vi "VIP_Pre-Install Custom Action.vi"(10 "Variant":variant) -> (0 "error out":errorcluster)   [LabVIEW 2020]
uses:
  <userlib>/_OpenG.lib/file/file.llb/openg_file.lvlib
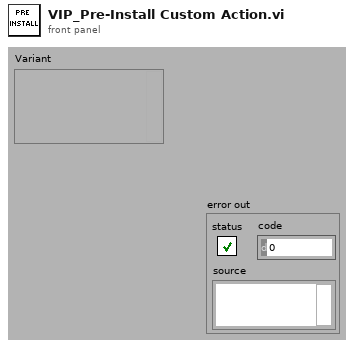
[diagram p1: front panel]
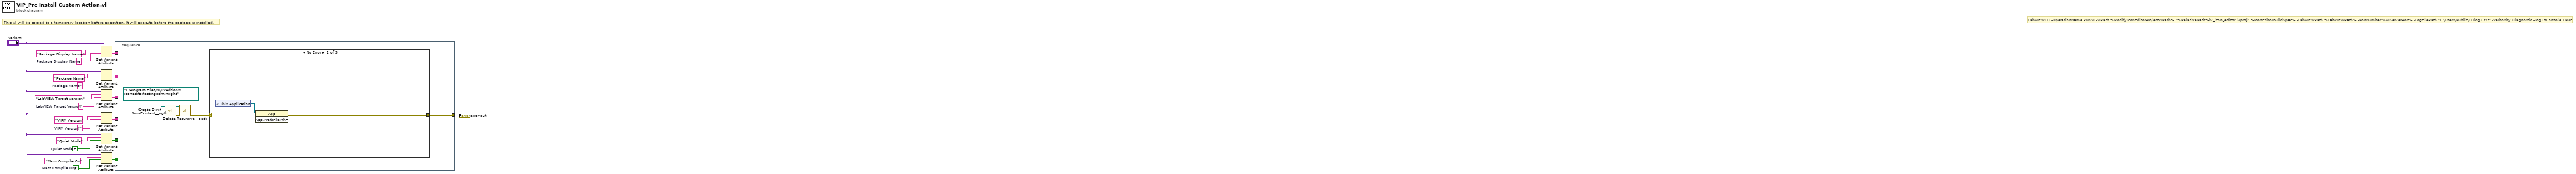
[diagram p0: block diagram]
diagram:
  w2 = FALSE  # Mass Compile On
  w4 = ""  # Package Display Name
  w11 = FALSE  # Quiet Mode
  w14 = ""  # VIPM Version
  w16 = ""  # LabVIEW Target Version
  w18 = ""  # Package Name
  # "LabVIEWCLI -OperationName RunVI -VIPath %ModifyIconEditorProjectVIPath% \"%RelativePath%lv_icon_editor.lvproj\" %IconEditorBuildSpec% -LabVIEWPath %LabVIEWPath% -PortNumber %VIServerPort% -LogFilePath \"C:\\Users\\Public\\CLIlog1.txt\" -Verbosity Diagnostic -LogToConsole TRUE"
  # "This VI will be copied to a temporary location before execution. It will execute before the package is installed."
  n1 = Get Variant Attribute(Variant="Variant", name="Package Display Name", default value (empty Variant)=w4) -> (value=w10:string)  [unwired: 1 in, 3 out]
  n2 = Get Variant Attribute(Variant="Variant", name="Package Name", default value (empty Variant)=w18) -> (value=w9:string)  [unwired: 1 in, 3 out]
  n3 = Get Variant Attribute(Variant="Variant", name="LabVIEW Target Version", default value (empty Variant)=w16) -> (value=w8:string)  [unwired: 1 in, 3 out]
  n4 = Get Variant Attribute(Variant="Variant", name="VIPM Version", default value (empty Variant)=w14) -> (value=w7:string)  [unwired: 1 in, 3 out]
  n5 = Get Variant Attribute(Variant="Variant", name="Quiet Mode", default value (empty Variant)=w11) -> (value=w6:bool)  [unwired: 1 in, 3 out]
  n6 = Get Variant Attribute(Variant="Variant", name="Mass Compile On", default value (empty Variant)=w2) -> (value=w5:bool)  [unwired: 1 in, 3 out]
  n7 = stacked-sequence {
    tunnel: w10 -> [_]
    tunnel: w9 -> [_]
    tunnel: w8 -> [_]
    tunnel: w7 -> [_]
    tunnel: w6 -> [_]
    tunnel: w5 -> [_]
    tunnel: [w25] -> w1
    frame #0 {
      n8 = call <userlib>:"Create Dir if Non-Existant__ogtk.vi"("Directory Path"=path "C:/Program Files/NI/LVAddons/iconeditortestingadminright" ("file path")) -> ("error out"=w23:errorcluster, "dup Directory Path"=w22:path)  [unwired: 8 in, 1 out]
      n9 = call <userlib>:"Delete Recursive__ogtk.vi"("error in (no error)"=w23, "Path"=w22) -> ("error out"=w24:errorcluster)  [unwired: 8 in, 1 out]
      n10 = case shown="No Error" w24 {
        selector: w24 -> [w26 _ w29]
        tunnel: [w26 w27 w29] -> w25
        frame Default {
        }
        frame No Error {
          n11 = control-ref of="This Application"() -> (w28:refnum<vi>)
          n12 = property class="App" props=["App.PrefsFilePth"](reference=w28) -> (error out=w27:errorcluster)  [unwired: 1 in, 2 out]
        }
        frame Error {
        }
      }
    }
  }
  "error out" <- w1
